vi "New.vi"(5 "Auto-generate TOC?":bool caption="Auto-generate TOC? (F)", 7 "Table of Contents?":bool caption="Table of Contents? (F)", 8 "error in (no error)":errorcluster, 9 "Default topic":string, 10 "Title":string, 11 "Base Path":path) -> (0 "error out":errorcluster, 3 "CHM Generator out":refnum<class "CHM Generator.lvclass">)   [LabVIEW 2027, in "CHM Generator.lvclass"]
uses:
  CHM Generator.lvclass
  CHM Generator.lvclass/CHM Generator.ctl
  Keyed Value Tree/Keyed Value Tree.lvclass
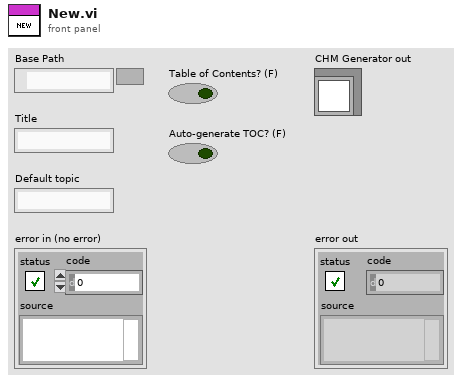
[diagram p1: front panel]
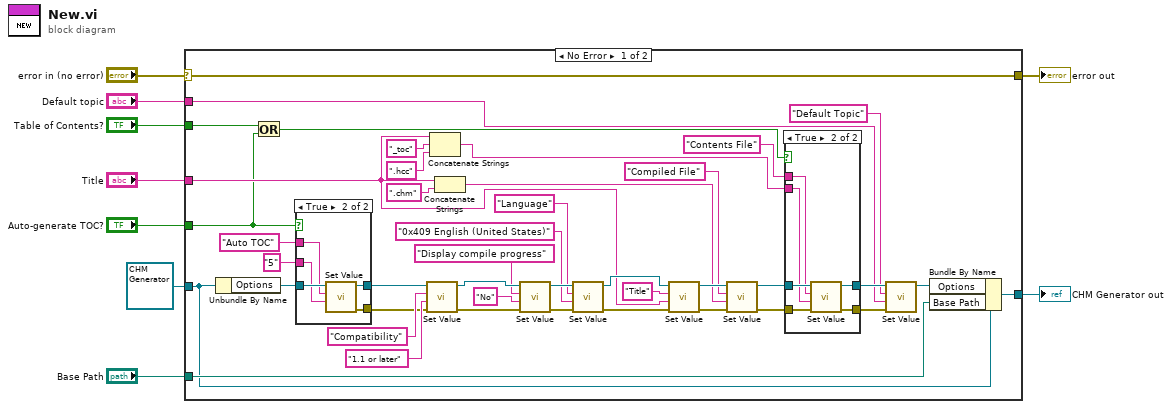
[diagram p0: block diagram]
diagram:
  n1 = case shown="No Error" "error in (no error)" {
    selector: "error in (no error)" -> [w51 w67]
    tunnel: [w51 w67] -> w8
    tunnel: [w26 w66] -> w6
    tunnel: refnum<class "CHM Generator.lvclass"> refnum ("CHM Generator in") -> [w16 w66]
    tunnel: "Default topic" -> [w28 _]
    tunnel: "Title" -> [w22 _]
    tunnel: "Base Path" -> [w20 _]
    tunnel: "Table of Contents?" -> [w18 _]
    tunnel: "Auto-generate TOC?" -> [w12 _]
    frame No Error {
      n2 = Unbundle By Name(w16) -> ("Options"=w15:refnum<class "Keyed Value Tree.lvclass">)
      n3 = Or(x=w18, y=w12) -> (x .or. y?=w17:bool)
      n4 = case shown="True" w12 {
        tunnel: w15 -> [w52 w57]
        tunnel: [w52 w56] -> w14
        tunnel: [_ w55] -> w13
        tunnel: "5" -> [_ w54]
        tunnel: "Auto TOC" ("name") -> [_ w53]
        frame False {
        }
        frame True {
          n5 = call-dynamic "Set Value.vi"("value"=w54, "name"=w53, "Keyed Value Tree in"=w57) -> ("error out"=w55:errorcluster, "Keyed Value Tree out"=w56:refnum<class "Keyed Value Tree.lvclass">)  [unwired: 6 in, 1 out]
        }
      }
      n6 = call-dynamic "Set Value.vi"("error in (no error)"=w13, "value"="1.1 or later", "name"="Compatibility", "Keyed Value Tree in"=w14) -> ("error out"=w47:errorcluster, "Keyed Value Tree out"=w48:refnum<class "Keyed Value Tree.lvclass">)  [unwired: 5 in, 1 out]
      n7 = Concatenate Strings(w22, "_toc" ("string"), ".hcc" ("string")) -> (w19:string)
      n8 = Concatenate Strings(w22, ".chm" ("string")) -> (w24:string)
      n9 = call-dynamic "Set Value.vi"("error in (no error)"=w47, "value"="No", "name"="Display compile progress", "Keyed Value Tree in"=w48) -> ("error out"=w44:errorcluster, "Keyed Value Tree out"=w43:refnum<class "Keyed Value Tree.lvclass">)  [unwired: 5 in, 1 out]
      n10 = call-dynamic "Set Value.vi"("error in (no error)"=w44, "value"="0x409 English (United States)", "name"="Language", "Keyed Value Tree in"=w43) -> ("error out"=w39:errorcluster, "Keyed Value Tree out"=w40:refnum<class "Keyed Value Tree.lvclass">)  [unwired: 5 in, 1 out]
      n11 = call-dynamic "Set Value.vi"("error in (no error)"=w39, "value"=w22, "name"="Title", "Keyed Value Tree in"=w40) -> ("error out"=w38:errorcluster, "Keyed Value Tree out"=w37:refnum<class "Keyed Value Tree.lvclass">)  [unwired: 5 in, 1 out]
      n12 = call-dynamic "Set Value.vi"("error in (no error)"=w38, "value"=w24, "name"="Compiled File", "Keyed Value Tree in"=w37) -> ("error out"=w36:errorcluster, "Keyed Value Tree out"=w35:refnum<class "Keyed Value Tree.lvclass">)  [unwired: 5 in, 1 out]
      n13 = case shown="True" w17 {
        tunnel: w36 -> [w58 w65]
        tunnel: w35 -> [w59 w64]
        tunnel: [w58 w63] -> w34
        tunnel: [w59 w62] -> w33
        tunnel: "Contents File" ("name") -> [_ w61]
        tunnel: w19 -> [_ w60]
        frame False {
        }
        frame True {
          n14 = call-dynamic "Set Value.vi"("error in (no error)"=w65, "value"=w60, "name"=w61, "Keyed Value Tree in"=w64) -> ("error out"=w63:errorcluster, "Keyed Value Tree out"=w62:refnum<class "Keyed Value Tree.lvclass">)  [unwired: 5 in, 1 out]
        }
      }
      n15 = call-dynamic "Set Value.vi"("error in (no error)"=w34, "value"=w28, "name"="Default Topic", "Keyed Value Tree in"=w33) -> ("Keyed Value Tree out"=w27:refnum<class "Keyed Value Tree.lvclass">)  [unwired: 5 in, 2 out]
      n16 = Bundle By Name(cluster=w16, "Options"=w27, "Base Path"=w20) -> (w26:refnum<class "CHM Generator.lvclass">)
    }
    frame Error {
    }
  }
  "error out" <- w8
  "CHM Generator out" <- w6
